vi "RSZVB Configure SAW Matching Network.vi"(4 "Parallel L (1.0e-9 H)":dbl=1e-09 format="%^.3e", 5 "Common Mode Impedance (25.0)":dbl=25.0 format="%^.3e", 6 "Differential Mode Impedance (100.0)":dbl=100.0 format="%^.3e", 7 "Serial C (1.0e-9 F)":dbl=1e-09 format="%^.3e", 8 "error in (no error)":errorcluster {"code" format="%.0x"}, 9 "Apply (F: Off)":bool, 10 "Channel (1)":i32=1, 11 "VISA session":refnum<visa-resource-name>) -> (0 "error out":errorcluster {"code" format="%.0x"}, 3 "dup VISA session":refnum<visa-resource-name>)   [LabVIEW 2011]
doc: "This VI configures SAW Matching Network parameters.\n\nRemote-control command(s):\nCALCulate<Ch>:FSIMulator:STATe ON | OFF\nCALCulate<Ch>:FSIMulator:BALun:DMCircuit:BPORt2:PARameters:L\nCALCulate<Ch>:FSIMulator:BALun:DMCircuit:BPORt2:PARameters:C\nCALCulate<Ch>:FSIMulator:BALun:DZConversion:BPORt2:ZDIFferent[:R]\nCALCulate<Ch>:FSIMulator:BALun:DZConversion:BPORt2:ZCOMmon[:R]"
panel:
  # "On\nOff"
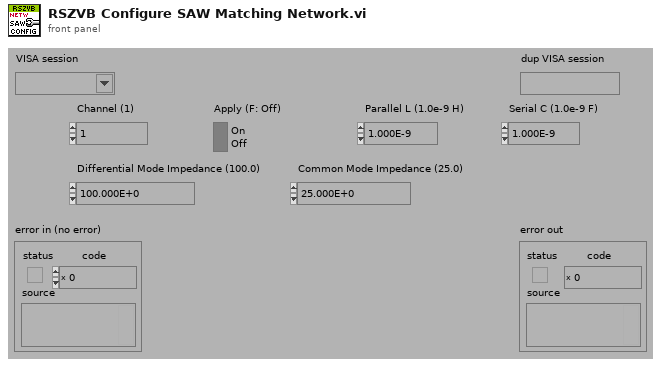
[diagram p1: front panel]
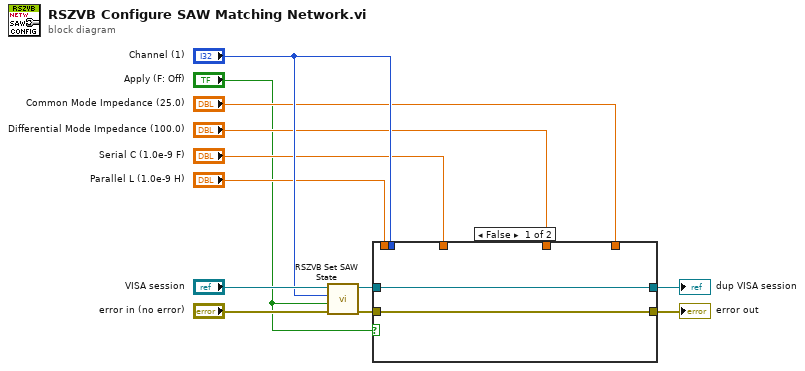
[diagram p0: block diagram]
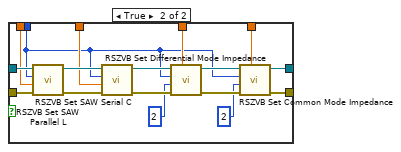
[diagram p2: hidden frame]
diagram:
  n1 = call "RSZVB Set SAW State.vi"("error in (no error)"="error in (no error)", "Apply (F: Off)"="Apply (F: Off)", "Channel (1)"="Channel (1)", "VISA session"="VISA session") -> ("error out"=w9:errorcluster, "dup VISA session"=w10:refnum<visa-resource-name>)  [unwired: 6 in]
  n2 = case shown="False" "Apply (F: Off)" {
    tunnel: [w13 w31] -> w12
    tunnel: [w14 w30] -> w11
    tunnel: w10 -> [w14 w29]
    tunnel: w9 -> [w13 w22]
    tunnel: "Channel (1)" -> [_ w15]
    tunnel: "Common Mode Impedance (25.0)" -> [_ w21]
    tunnel: "Differential Mode Impedance (100.0)" -> [_ w20]
    tunnel: "Serial C (1.0e-9 F)" -> [_ w19]
    tunnel: "Parallel L (1.0e-9 H)" -> [_ w18]
    frame False {
    }
    frame True {
      n3 = call "RSZVB Set SAW Parallel L.vi"("error in (no error)"=w22, "Parallel L (1.0e-9 H)"=w18, "Channel (1)"=w15, "VISA session"=w29) -> ("error out"=w23:errorcluster, "dup VISA session"=w28:refnum<visa-resource-name>)  [unwired: 6 in]
      n4 = call "RSZVB Set SAW Serial C.vi"("error in (no error)"=w23, "Serial C (1.0e-9 F)"=w19, "Channel (1)"=w15, "VISA session"=w28) -> ("error out"=w24:errorcluster, "dup VISA session"=w27:refnum<visa-resource-name>)  [unwired: 6 in]
      n5 = call "RSZVB Set Differential Mode Impedance.vi"("Impedance (100)"=w20, "error in (no error)"=w24, "Logical Port (1)"=2, "Channel (1)"=w15, "VISA session"=w27) -> ("error out"=w25:errorcluster, "dup VISA session"=w26:refnum<visa-resource-name>)  [unwired: 5 in]
      n6 = call "RSZVB Set Common Mode Impedance.vi"("Impedance (25)"=w21, "error in (no error)"=w25, "Logical Port (1)"=2, "Channel (1)"=w15, "VISA session"=w26) -> ("error out"=w31:errorcluster, "dup VISA session"=w30:refnum<visa-resource-name>)  [unwired: 5 in]
    }
  }
  "error out" <- w12
  "dup VISA session" <- w11
